vi "camara.vi"() -> ()   [LabVIEW 2010]
uses:
  <vilib>/addons/PixeLINK/Low Level Functions/ERROR_REPORTING.llb/TDPU-ErrorReporting-Error_Report.ctl
  <vilib>/addons/PixeLINK/Low Level Functions/CAMERA_FEATURES.llb/TDPU-CameraFeatures-PixelFormat.ctl
  <vilib>/addons/PixeLINK/Low Level Functions/TRANSLATION.llb/TDPU-Translation-ImageFileFormat.ctl
  <vilib>/addons/PixeLINK/Low Level Functions/ACQUISITION.llb/TDPU-Acquisition-StreamState.ctl
  <vilib>/addons/PixeLINK/Low Level Functions/CAMERA_FEATURES.llb/TDPU-CameraFeatures-FeatureIds.ctl
  <vilib>/addons/PixeLINK/Low Level Functions/CAMERA_FEATURES.llb/TDPU-CameraFeatures-FeatureFlags.ctl
panel:
  out "*(type *) &x":u16[](array[numeric])
  out "Width":dbl
  out "Height":dbl
  out "Image 2":T1(plugin-control)
  out "error out 2":errorcluster
  in  "error in (no error) 2":errorcluster
  out "Raw Output PIXEL_FORMAT":T2 items=["PIXEL_FORMAT_MONO8", "PIXEL_FORMAT_MONO16", "PIXEL_FORMAT_YUV422", "PIXEL_FORMAT_BAYER8_GRBG", "PIXEL_FORMAT_BAYER16_GRBG", "PIXEL_FORMAT_RGB24", "PIXEL_FORMAT_RGB48", "PIXEL_FORMAT_BAYER8_RGGB", "PIXEL_FORMAT_BAYER8_GBRG ", "PIXEL_FORMAT_BAYER8_BGGR ", "PIXEL_FORMAT_BAYER16_RGGB ", "PIXEL_FORMAT_BAYER16_GBRG", "PIXEL_FORMAT_BAYER16_BGGR", "PIXEL_FORMAT_RGB32"]
  in  "IMAGE_FILE_FORMAT":T3=4 items=["IMAGE_FORMAT_BMP", "IMAGE_FORMAT_TIFF", "IMAGE_FORMAT_PSD", "IMAGE_FORMAT_JPEG", "IMAGE_FORMAT_RAW_RGB24", "IAMGE_FORMAT_RAW_RGB32"]
  in  "Requested PIXEL_FORMAT":T2 items=["PIXEL_FORMAT_MONO8", "PIXEL_FORMAT_MONO16", "PIXEL_FORMAT_YUV422", "PIXEL_FORMAT_BAYER8_GRBG", "PIXEL_FORMAT_BAYER16_GRBG", "PIXEL_FORMAT_RGB24", "PIXEL_FORMAT_RGB48", "PIXEL_FORMAT_BAYER8_RGGB", "PIXEL_FORMAT_BAYER8_GBRG ", "PIXEL_FORMAT_BAYER8_BGGR ", "PIXEL_FORMAT_BAYER16_RGGB ", "PIXEL_FORMAT_BAYER16_GBRG", "PIXEL_FORMAT_BAYER16_BGGR", "PIXEL_FORMAT_RGB32"]
  out "pLVErrorReport OUT":T4 {"uReturnCode" format="%.0x"}
  in  "Stop App":bool
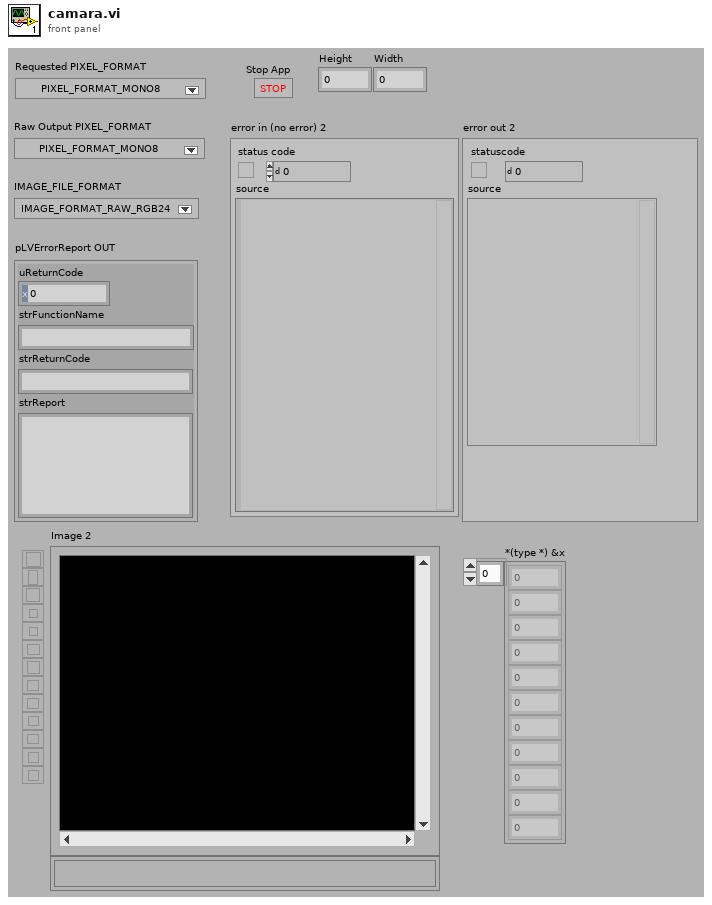
[diagram p1: front panel]
types:
  T1 = typedef "IMAQ Image.ctl" = refnum<image>
  T2 = typedef "TDPU-CameraFeatures-PixelFormat.ctl" = u16
  T3 = typedef "TDPU-Translation-ImageFileFormat.ctl" = u32
  T4 = typedef "TDPU-ErrorReporting-Error_Report.ctl" = cluster{"uReturnCode":i32, "strFunctionName":string, "strReturnCode":string, "strReport":string}
  T5 = typedef "TDPU-Acquisition-StreamState.ctl" = u32
  T6 = typedef "TDPU-CameraFeatures-FeatureIds.ctl" = u32
  T7 = typedef "TDPU-Acquisition-Frame_Desc.ctl" = cluster{"uSize":u32, "fFrameTime":dbl, "uFrameNumber":u32, "Brightness":cluster{"fValue":dbl}, "AutoExposure":cluster{"fValue":dbl}, "Sharpness":cluster{"fValue":dbl}, "WhiteBalance":cluster{"fValue":dbl}, "Hue":cluster{"fValue":dbl}, "Saturation":cluster{"fValue":dbl}, "Gamma":cluster{"fValue":dbl}, "Shutter":cluster{"fValue":dbl}, "Gain":cluster{"fValue":dbl}, "Iris":cluster{"fValue":dbl}, "Focus":cluster{"fValue":dbl}, "Temperature":cluster{"fValue":dbl}, "Trigger":cluster{"fMode":dbl, "fType":dbl, "fPolarity":dbl, "fDelay":dbl, "fParameter":dbl}, "Zoom":cluster{"fValue":dbl}, "Pan":cluster{"fValue":dbl}, "Tilt":cluster{"fValue":dbl}, "OpticalFilter":cluster{"fValue":dbl}, "GPIO":cluster{"fMode":dbl[], "fPolarity":dbl[], "fParameter1":dbl[], "fParameter2":dbl[], "fParameter3":dbl[]}, "FrameRate":cluster{"fValue":dbl}, "ROI":cluster{"fLeft":dbl, "fTop":dbl, "fWidth":dbl, "fHeight":dbl}, "Flip":cluster{"fHorizontal":dbl, "fVertical":dbl}, "PixelAddressingValue":cluster{"fValue":dbl}, "PixelFormat":cluster{"fValue":dbl}, "ExtendedShutter":cluster{"fKneePoint":dbl[]}, "AutoROI":cluster{"fLeft":dbl, "fTop":dbl, "fWidth":dbl, "fHeight":dbl}, "WhiteShading":cluster{"fRedGain":dbl, "fGreenGain":dbl, "fBlueGain":dbl}, "Rotate":cluster{"fValue":dbl}, "PixelAddressingMode":cluster{"fValue":dbl}}
  T8 = typedef "TDPU-CameraFeatures-FeatureFlags.ctl" = u32
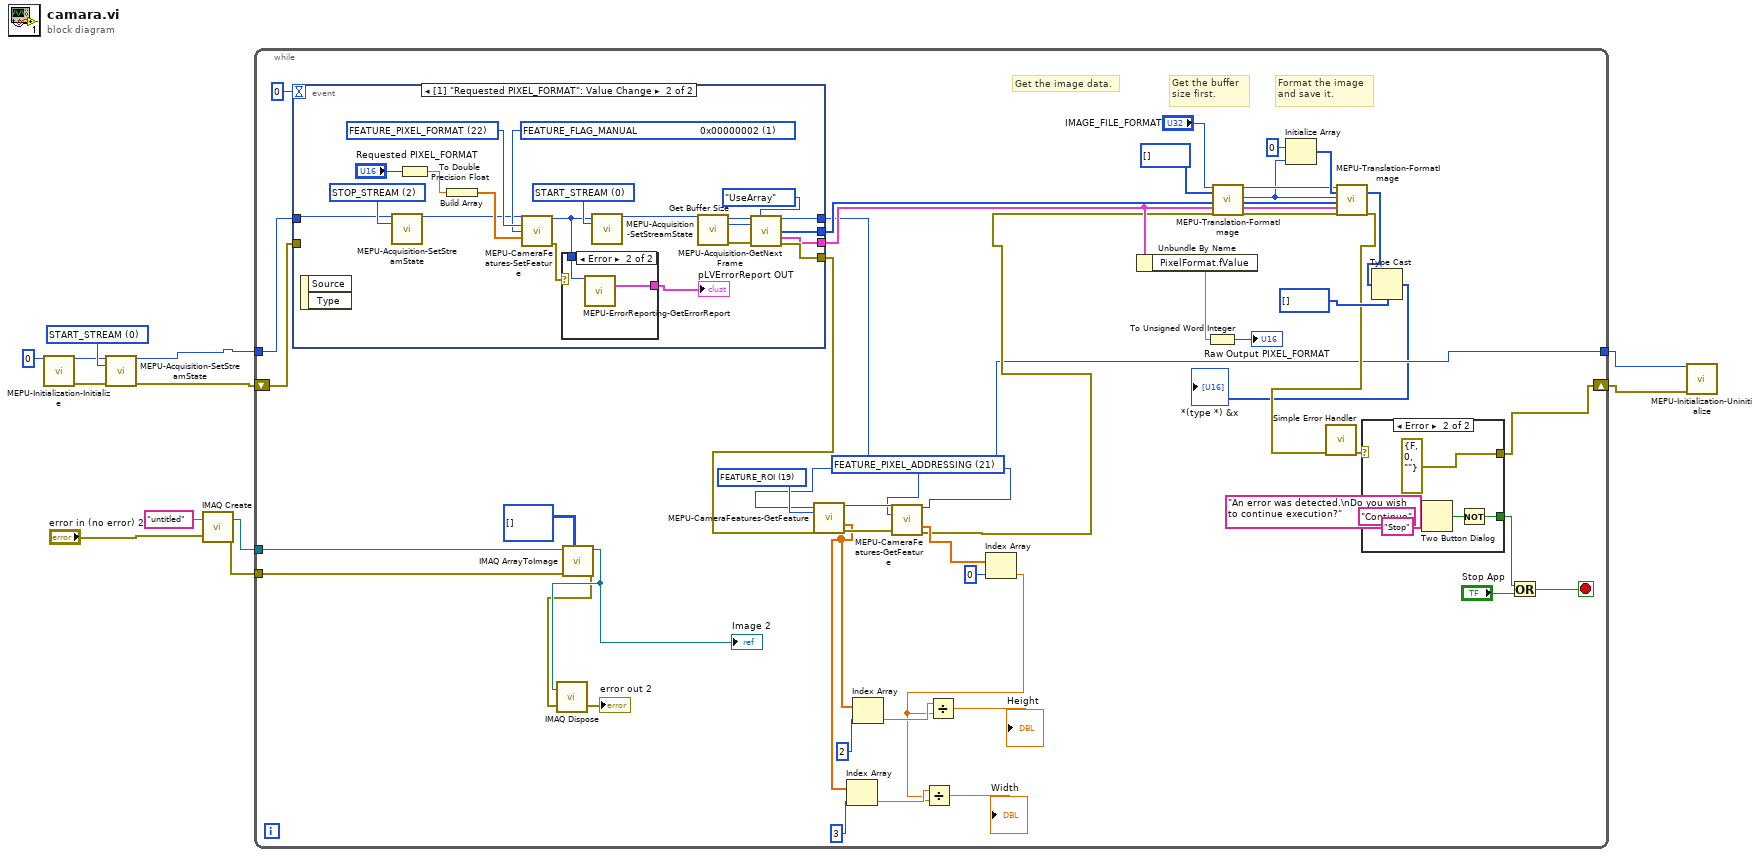
[diagram p0: block diagram]
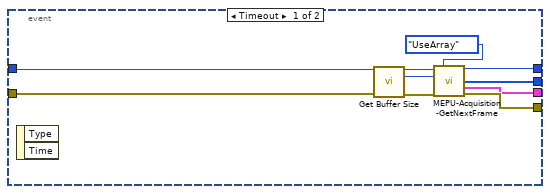
[diagram p2: hidden frame]
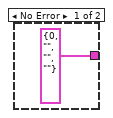
[diagram p3: hidden frame]
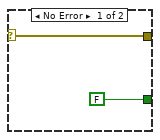
[diagram p4: hidden frame]
diagram:
  w11 = T5 0 items=["START_STREAM", "PAUSE_STREAM", "STOP_STREAM"] ("uStreamState IN")
  n1 = call <vilib>:"MEPU-Initialization-Initialize.vi"("uSerialNumber IN"=u32 0) -> ("phCamera OUT"=w9:u32, "Error OUT"=w8:errorcluster)  [unwired: 1 in, 12 out]
  n2 = call <vilib>:"MEPU-Acquisition-SetStreamState.vi"("hCamera IN"=w9, "uStreamState IN"=w11, "Error IN"=w8) -> ("hCamera OUT"=w6:u32, "Error OUT"=w7:errorcluster)  [unwired: 11 out]
  n3 = call "IMAQ Create"("Image Name"="untitled", "error in (no error)"="error in (no error) 2") -> ("New Image"=w2:T1, "error out"=w1:errorcluster)  [unwired: 3 in]
  n4 = while {
    tunnel: w6 -> [w57]
    tunnel: [w20] -> w12
    shift-right: [w38] -> w5
    shift-left: w7 -> [w56]
    tunnel: w2 -> [w37]
    tunnel: w1 -> [w36]
    stop <- w58 stop-if-true
    w29 = T6 21 items=["FEATURE_BRIGHTNESS", "FEATURE_EXPOSURE", "FEATURE_SHARPNESS", "FEATURE_WHITE_BAL", "FEATURE_HUE", "FEATURE_SATURATION", "FEATURE_GAMMA", "FEATURE_SHUTTER", "FEATURE_GAIN", "FEATURE_IRIS", "FEATURE_FOCUS", "FEATURE_TEMPERATURE", "FEATURE_TRIGGER", "FEATURE_ZOOM", "FEATURE_PAN", "FEATURE_TILT", "FEATURE_OPT_FILTER", "FEATURE_GPIO", "FEATURE_FRAME_RATE", "FEATURE_ROI", "FEATURE_FLIP", "FEATURE_PIXEL_ADDRESSING", "FEATURE_PIXEL_FORMAT", "FEATURE_EXTENDED_SHUTTER", "FEATURE_AUTO_ROI", "FEATURE_LOOKUP_TABLE", "FEATURE_MEMORY_CHANNEL", "FEATURE_WHITE_SHADING", "FEATURE_ROTATE", "FEATURE_IMAGER_CLK_DIVISOR", "FEATURE_TRIG_WITH_CNTRLD_LIGHT", "FEATURE_MAX_PIXEL_SIZE"] ("uFeatureId IN")
    w33 = T6 19 items=["FEATURE_BRIGHTNESS", "FEATURE_EXPOSURE", "FEATURE_SHARPNESS", "FEATURE_WHITE_BAL", "FEATURE_HUE", "FEATURE_SATURATION", "FEATURE_GAMMA", "FEATURE_SHUTTER", "FEATURE_GAIN", "FEATURE_IRIS", "FEATURE_FOCUS", "FEATURE_TEMPERATURE", "FEATURE_TRIGGER", "FEATURE_ZOOM", "FEATURE_PAN", "FEATURE_TILT", "FEATURE_OPT_FILTER", "FEATURE_GPIO", "FEATURE_FRAME_RATE", "FEATURE_ROI", "FEATURE_FLIP", "FEATURE_PIXEL_ADDRESSING", "FEATURE_PIXEL_FORMAT", "FEATURE_EXTENDED_SHUTTER", "FEATURE_AUTO_ROI", "FEATURE_LOOKUP_TABLE", "FEATURE_MEMORY_CHANNEL", "FEATURE_WHITE_SHADING", "FEATURE_ROTATE", "FEATURE_IMAGER_CLK_DIVISOR", "FEATURE_TRIG_WITH_CNTRLD_LIGHT", "FEATURE_MAX_PIXEL_SIZE"] ("uFeatureId IN")
    # "Format the image\nand save it."
    # "Get the image data."
    # "Get the buffer \nsize first."
    n5 = event shown="[1] \"Requested PIXEL_FORMAT\": Value Change" {
      selector: _ -> [_ _]
      dyn-events: _ -> [_ _]
      timeout: 0 -> [_ _]
      tunnel: w57 -> [w62 w86]
      tunnel: w56 -> [w63 _]
      tunnel: [w70 w76] -> w22
      tunnel: [w71 w75] -> w23
      tunnel: [w68 w74] -> w42
      tunnel: [w69 w73] -> w41
      event Timeout {
        n6 = event-data() -> ()  [unwired: 3 out]
        n7 = call "Get Buffer Size.vi"("phCamera IN"=w62, "Error IN"=w63) -> ("phCamera OUT"=w67:u32, "uBufferSize OUT"=w65:u32, "Error OUT"=w64:errorcluster)  [unwired: 11 out]
        n8 = call <vilib>:"MEPU-Acquisition-GetNextFrame.vi"("hCamera IN"=w67, "Mode IN"=enum16{"UseArray", "UsePointer"}."UseArray", "uBufferSize IN"=w65, "Error IN"=w64) -> ("hCamera OUT"=w71:u32, "Data OUT"=w68:u8[], "pDescriptor"=w69:T7, "Error OUT"=w70:errorcluster)  [unwired: 2 in, 6 out]
      }
      event Value Change {
        w84 = T5 0 items=["START_STREAM", "PAUSE_STREAM", "STOP_STREAM"] ("uStreamState IN")
        w87 = T5 2 items=["START_STREAM", "PAUSE_STREAM", "STOP_STREAM"] ("uStreamState IN")
        w91 = T8 1 items=["FEATURE_FLAG_PRESENCE                 0x00000001", "FEATURE_FLAG_MANUAL                     0x00000002", "FEATURE_FLAG_AUTO                         0x00000004", "FEATURE_FLAG_ONEPUSH                   0x00000008", "FEATURE_FLAG_OFF                            0x00000010", "FEATURE_FLAG_DESC_SUPPORTED    0x00000020", "FEATURE_FLAG_READ_ONLY               0x00000040"] ("uFlags IN")
        w92 = T6 22 items=["FEATURE_BRIGHTNESS", "FEATURE_EXPOSURE", "FEATURE_SHARPNESS", "FEATURE_WHITE_BAL", "FEATURE_HUE", "FEATURE_SATURATION", "FEATURE_GAMMA", "FEATURE_SHUTTER", "FEATURE_GAIN", "FEATURE_IRIS", "FEATURE_FOCUS", "FEATURE_TEMPERATURE", "FEATURE_TRIGGER", "FEATURE_ZOOM", "FEATURE_PAN", "FEATURE_TILT", "FEATURE_OPT_FILTER", "FEATURE_GPIO", "FEATURE_FRAME_RATE", "FEATURE_ROI", "FEATURE_FLIP", "FEATURE_PIXEL_ADDRESSING", "FEATURE_PIXEL_FORMAT", "FEATURE_EXTENDED_SHUTTER", "FEATURE_AUTO_ROI", "FEATURE_LOOKUP_TABLE", "FEATURE_MEMORY_CHANNEL", "FEATURE_WHITE_SHADING", "FEATURE_ROTATE", "FEATURE_IMAGER_CLK_DIVISOR", "FEATURE_MAX_PIXEL_SIZE", "FEATURE_TRIG_WITH_CNTRLD_LIGHT"] ("uFeatureId IN")
        n9 = event-data() -> ()  [unwired: 3 out]
        n10 = call <vilib>:"MEPU-Acquisition-SetStreamState.vi"("hCamera IN"=w86, "uStreamState IN"=w87) -> ("hCamera OUT"=w85:u32)  [unwired: 1 in, 12 out]
        n11 = To Double Precision Float(number="Requested PIXEL_FORMAT") -> (double precision float=w89:dbl)
        n12 = Build Array(w89) -> (w88:dbl[])
        n13 = call <vilib>:"MEPU-CameraFeatures-SetFeature.vi"("hCamera IN"=w85, "uFeatureId IN"=w92, "uFlags IN"=w91, "pParms IN"=w88) -> ("hCamera OUT"=w81:u32, "Error OUT"=w72:errorcluster)  [unwired: 1 in, 9 out]
        n14 = case shown="Error" w72 {
          tunnel: [T4 {"uReturnCode"=0, "strFunctionName"="", "strReturnCode"="", "strReport"=""} ("pLVErrorReport OUT") w95] -> w82
          tunnel: w81 -> [_ w94]
          frame No Error {
          }
          frame Error {
            n15 = call <vilib>:"MEPU-ErrorReporting-GetErrorReport.vi"("hCamera IN"=w94) -> ("pLVErrorReport OUT"=w95:T4)  [unwired: 1 in, 13 out]
          }
        }
        "pLVErrorReport OUT" <- w82
        n16 = call <vilib>:"MEPU-Acquisition-SetStreamState.vi"("hCamera IN"=w81, "uStreamState IN"=w84) -> ("hCamera OUT"=w83:u32)  [unwired: 1 in, 12 out]
        n17 = call "Get Buffer Size.vi"("phCamera IN"=w83) -> ("phCamera OUT"=w79:u32, "uBufferSize OUT"=w78:u32, "Error OUT"=w77:errorcluster)  [unwired: 1 in, 11 out]
        n18 = call <vilib>:"MEPU-Acquisition-GetNextFrame.vi"("hCamera IN"=w79, "Mode IN"=enum16{"UseArray", "UsePointer"}."UseArray", "uBufferSize IN"=w78, "Error IN"=w77) -> ("hCamera OUT"=w75:u32, "Data OUT"=w74:u8[], "pDescriptor"=w73:T7, "Error OUT"=w76:errorcluster)  [unwired: 2 in, 6 out]
      }
    }
    n19 = call "IMAQ ArrayToImage"("Image Pixels (U16)"=u16[][] [], "error in (no error)"=w36, "Image"=w37) -> ("error out"=w15:errorcluster, "Image Out"=w16:T1)  [unwired: 7 in]
    "Image 2" <- w16
    n20 = call "IMAQ Dispose"("Image"=w16, "error in (no error)"=w15) -> ("error out"=→"error out 2":errorcluster)  [unwired: 4 in]
    n21 = call <vilib>:"MEPU-CameraFeatures-GetFeature.vi"("hCamera IN"=w23, "uFeatureId IN"=w33, "Error IN"=w22) -> ("hCamera OUT"=w35:u32, "pParms OUT"=w30:dbl[], "Error OUT"=w34:errorcluster)  [unwired: 8 in, 2 out]
    n22 = Index Array(array=w30, index=3) -> (element=w25:dbl)
    n23 = Index Array(array=w30, index=2) -> (element=w26:dbl)
    n24 = call <vilib>:"MEPU-CameraFeatures-GetFeature.vi"("hCamera IN"=w35, "uFeatureId IN"=w29, "Error IN"=w34) -> ("hCamera OUT"=w20:u32, "pParms OUT"=w28:dbl[], "Error OUT"=w21:errorcluster)  [unwired: 8 in, 2 out]
    n25 = Index Array(array=w28, index=0) -> (element=w24:dbl)
    n26 = Divide(x=w25, y=w24) -> (x/y=→"Width":dbl)
    n27 = Divide(x=w26, y=w24) -> (x/y=→"Height":dbl)
    n28 = Unbundle By Name(w41) -> ("PixelFormat.fValue"=w46:dbl)
    n29 = To Unsigned Word Integer(number=w46) -> (unsigned 16bit integer=→"Raw Output PIXEL_FORMAT":u16)
    n30 = call <vilib>:"MEPU-Translation-FormatImage.vi"("uOutputFormat IN"="IMAGE_FILE_FORMAT", "pDest IN"=u8[] [], "pSrc IN"=w42, "pFrameDesc IN"=w41, "Error IN"=w21) -> ("uOutputFormat OUT"=w48:T3, "DestBufferSize OUT"=w47:u32, "pSrc OUT"=w51:u8[], "pFrameDesc OUT"=w50:T7, "Error OUT"=w54:errorcluster)  [unwired: 1 in, 9 out]
    n31 = Initialize Array(u8 0 ("element"), w47) -> (w49:u8[])
    n32 = call <vilib>:"MEPU-Translation-FormatImage.vi"("uOutputFormat IN"=w48, "pDest IN"=w49, "DestBufferSize IN"=w47, "pSrc IN"=w51, "pFrameDesc IN"=w50, "Error IN"=w54) -> ("pDest OUT"=w44:u8[], "Error OUT"=w40:errorcluster)  [unwired: 12 out]
    n33 = call <vilib>:"Simple Error Handler.vi"("error in (no error)"=w40) -> ("error out"=w61:errorcluster)  [unwired: 1 in, 7 out]
    n34 = case shown="Error" w61 {
      selector: w61 -> [w97 _]
      tunnel: [w97 errorcluster {"status"=FALSE, "code"=0, "source"=""} ("error IO")] -> w38
      tunnel: [FALSE ("T button?") w98] -> w60
      frame No Error {
      }
      frame Error {
        n35 = Two Button Dialog(message="An error was detected.\nDo you wish to continue execution?", 1:"Stop" ("F button name (\"Cancel\")"), 2:"Continue" ("T button name (\"OK\")")) -> (T button?=w99:bool)
        n36 = Not(x=w99) -> (.not. x?=w98:bool)
      }
    }
    n37 = Type Cast(type=u16[] [], x=w44) -> (*(type *) &x=→"*(type *) &x":u16[])
    n38 = Or(x=w60, y="Stop App") -> (x .or. y?=w58:bool)
  }
  n39 = call <vilib>:"MEPU-Initialization-Uninitialize.vi"("hCamera IN"=w12, "Error IN"=w5) -> ()  [unwired: 14 out]
